vi "CalculateTangentPoint.vi"(0 "object in":refnum<class "KickTactic.lvclass">, 5 "error in (no error)":errorcluster) -> (14 "object out":refnum<class "KickTactic.lvclass">, 19 "error out":errorcluster)   [LabVIEW 2023, in "KickTactic.lvclass"]
uses:
  KickTactic.lvclass
  KickTactic.lvclass/KickTactic.ctl
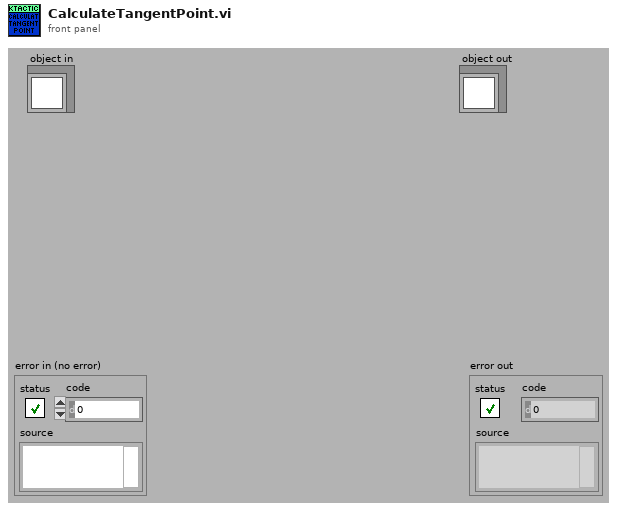
[diagram p1: front panel]
types:
  T1 = typedef "KickTactic.lvclass/KickTactic_states.ctl" = enum16{"GoToTangentPoint\n", "Circulate\n", "Align\n", "Kick\n", "Exit"}
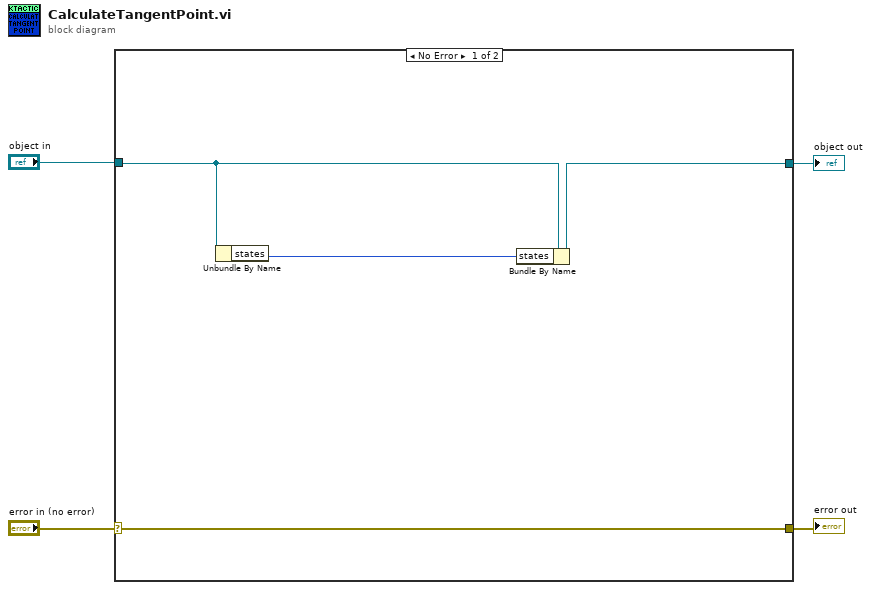
[diagram p0: block diagram]
diagram:
  n1 = case shown="No Error" "error in (no error)" {
    selector: "error in (no error)" -> [w7 w10]
    tunnel: [w7 w10] -> w3
    tunnel: [w5 w9] -> w1
    tunnel: "object in" -> [w6 w9]
    frame No Error {
      n2 = Unbundle By Name(w6) -> ("states"=w8:T1)
      n3 = Bundle By Name(cluster=w6, "states"=w8) -> (w5:refnum<class "KickTactic.lvclass">)
    }
    frame Error {
    }
  }
  "error out" <- w3
  "object out" <- w1
